vi "Windspeed Warning.vi"() -> ()   [LabVIEW 2017]
uses:
  Weather Data.ctl
panel:
  out "Error Out":errorcluster
  in  "Error In":errorcluster
  out "Weather Data In. 2":T1={"Current Temperature"=0.0, "Max Temperature"=0.0, "Min Temperature"=0.0, "Warning Text"="No Warning", "Temperature Warning?"=FALSE, "Enum"=enum."", "Current Windapeed"=0.0, "Max Windspeed"=0.0, "Windspeed Warning?"=FALSE, "Windspeed Warning text"=""}
  in  "Weather Data In.":T1={"Current Temperature"=0.0, "Max Temperature"=0.0, "Min Temperature"=0.0, "Warning Text"="No Warning", "Temperature Warning?"=FALSE, "Enum"=enum."", "Current Windapeed"=0.0, "Max Windspeed"=0.0, "Windspeed Warning?"=FALSE, "Windspeed Warning text"=""}
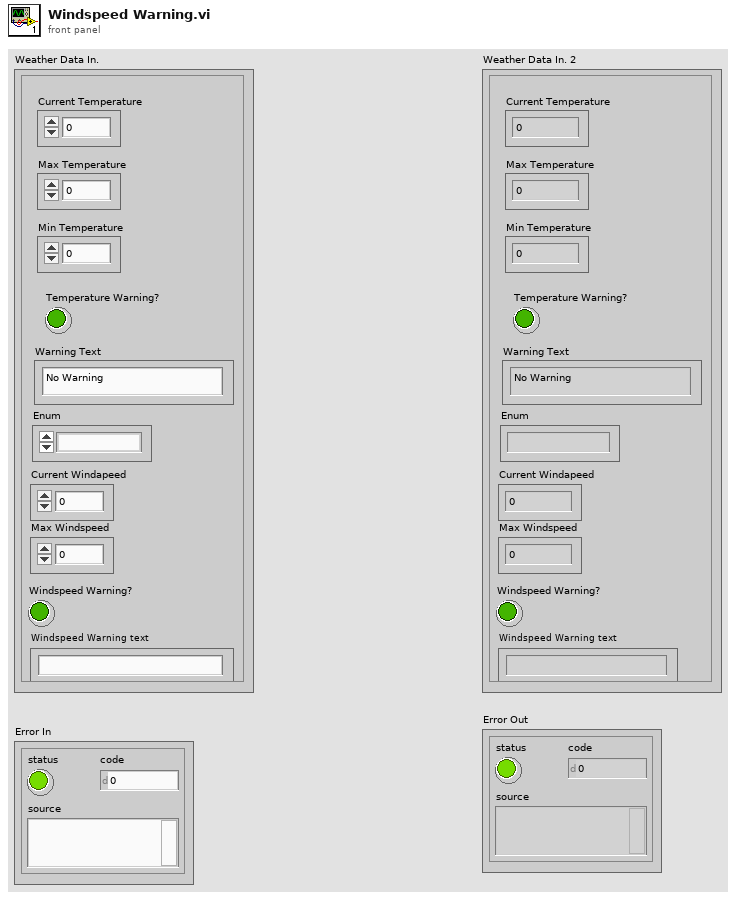
[diagram p1: front panel]
types:
  T1 = typedef "Weather Data.ctl" = cluster{"Current Temperature":dbl, "Max Temperature":dbl, "Min Temperature":dbl, "Warning Text":string, "Temperature Warning?":bool, "Enum":enum16{""}, "Current Windapeed":dbl, "Max Windspeed":dbl, "Windspeed Warning?":bool, "Windspeed Warning text":string}
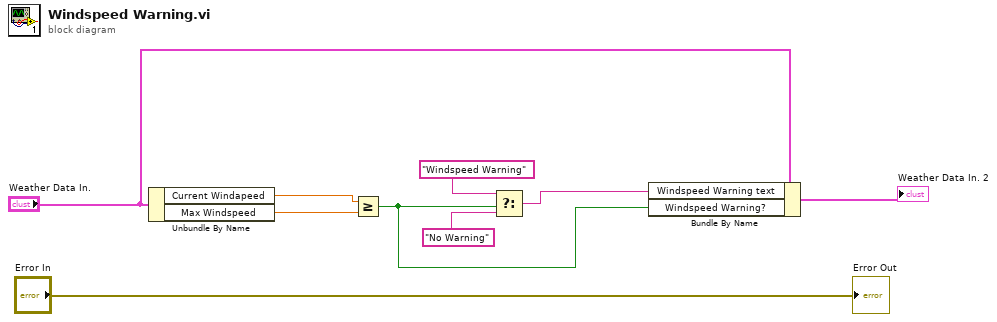
[diagram p0: block diagram]
diagram:
  n1 = Unbundle By Name("Weather Data In.") -> ("Current Windapeed"=w8:dbl, "Max Windspeed"=w7:dbl)
  n2 = Greater Or Equal?(x=w8, y=w7) -> (x >= y?=w2:bool)
  n3 = Select(t="Windspeed Warning", s=w2, f="No Warning") -> (s? t:f=w1:string)
  n4 = Bundle By Name(cluster="Weather Data In.", "Windspeed Warning text"=w1, "Windspeed Warning?"=w2) -> (→"Weather Data In. 2":T1)
  "Error Out" <- "Error In"
